vi "findMinimumValueInArray.vi"(8 "error in (no error)":errorcluster, 10 "array":i32[](array[numeric]), 11 "Utilities in":refnum<class "Utilities.lvclass">) -> (0 "error out":errorcluster, 2 "minimum":i32, 3 "Utilities out":refnum<class "Utilities.lvclass">)   [LabVIEW 2020, in "Utilities.lvclass"]
uses:
  Utilities.lvclass
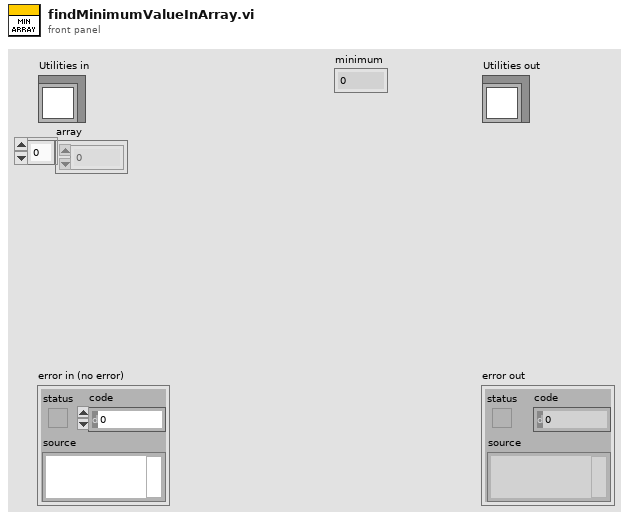
[diagram p1: front panel]
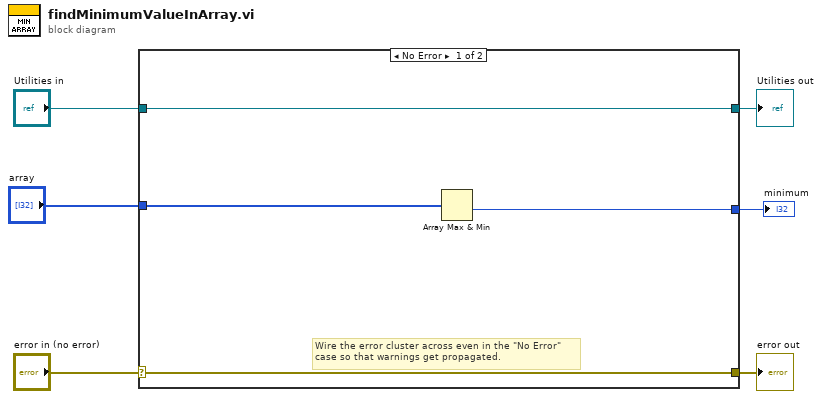
[diagram p0: block diagram]
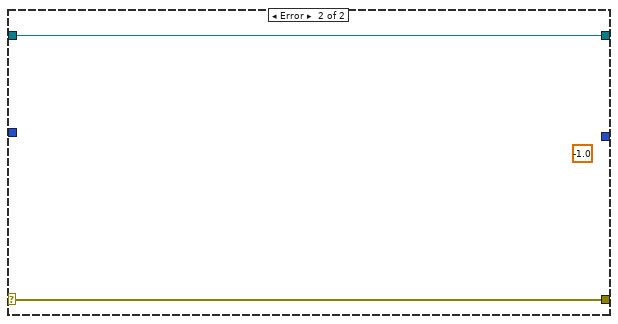
[diagram p2: hidden frame]
diagram:
  n1 = case shown="No Error" "error in (no error)" {
    selector: "error in (no error)" -> [w9 w12]
    tunnel: [w9 w12] -> w5
    tunnel: [w10 w11] -> w3
    tunnel: "Utilities in" -> [w10 w11]
    tunnel: "array" -> [w8 _]
    tunnel: [w7 _] -> w1
    frame No Error {
      # "Wire the error cluster across even in the \"No Error\"\ncase so that warnings get propagated."
      n2 = Array Max & Min(array=w8) -> (min value=w7:i32)  [unwired: 3 out]
    }
    frame Error {
      (unwired) -1.0
    }
  }
  "error out" <- w5
  "Utilities out" <- w3
  "minimum" <- w1
